vi "ClassifyRX.vi"(8 "error in (no error)":errorcluster, 10 "msg to Log":string, 11 "Log in":refnum<class "Log.lvclass">) -> (0 "error out":errorcluster, 3 "Log out":refnum<class "Log.lvclass">)   [LabVIEW 2018, in "Log.lvclass"]
uses:
  Log.lvclass
  Log.lvclass/Log.ctl
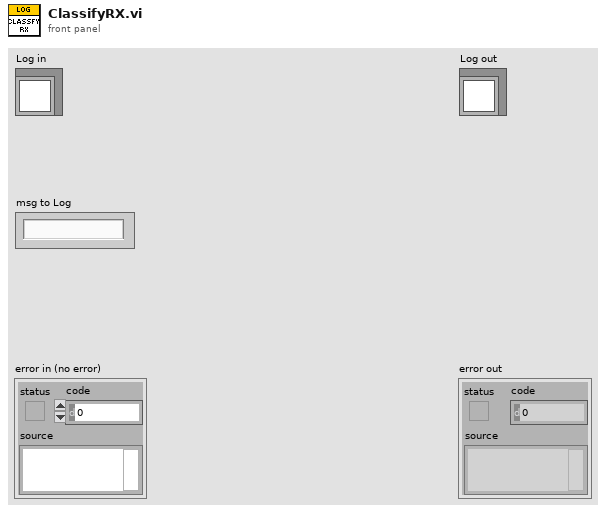
[diagram p1: front panel]
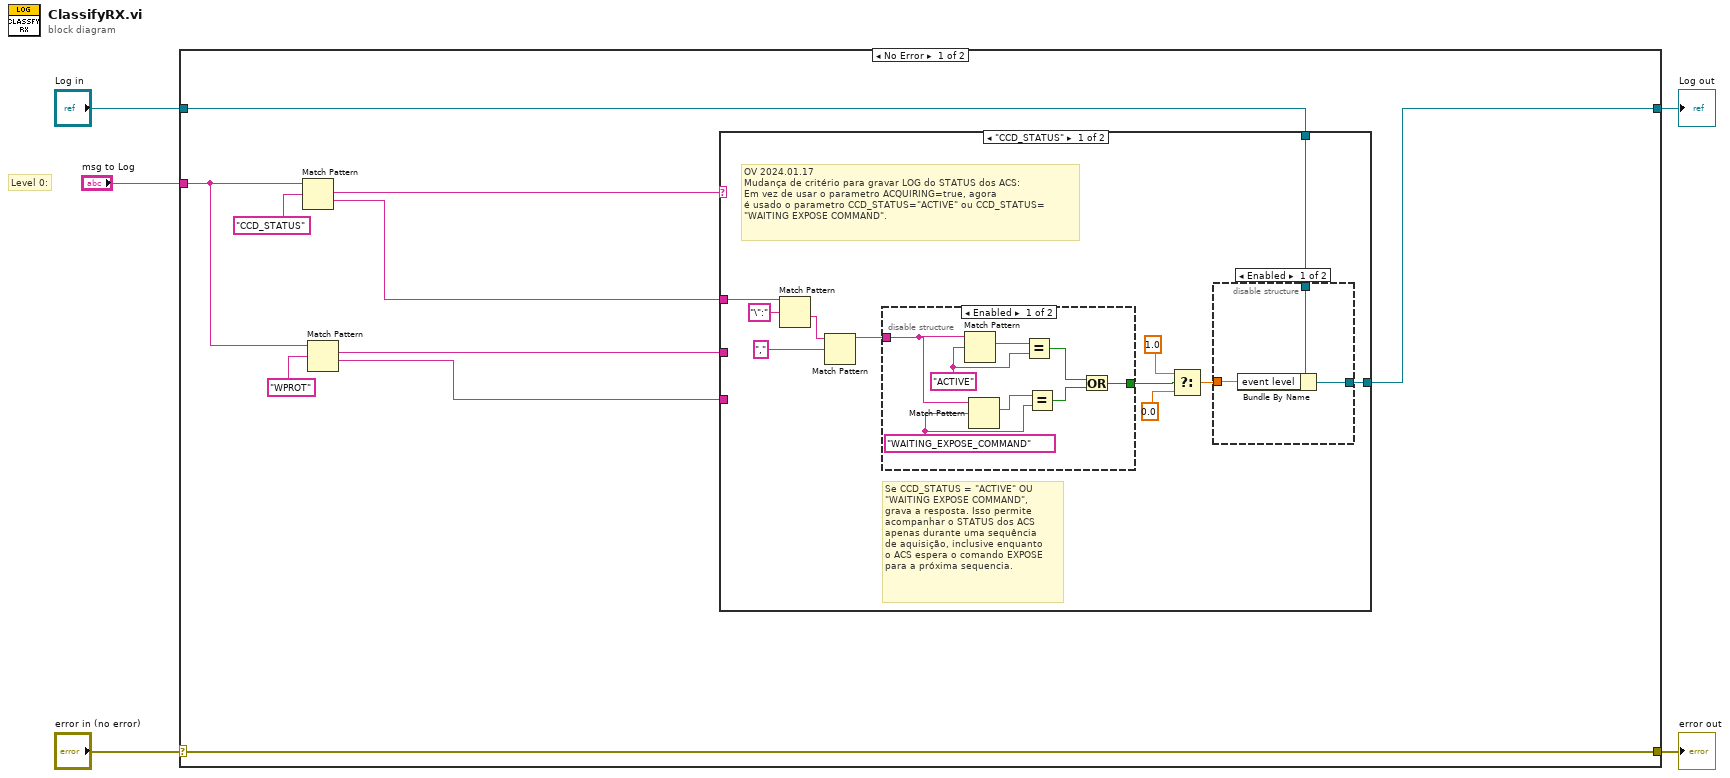
[diagram p0: block diagram]
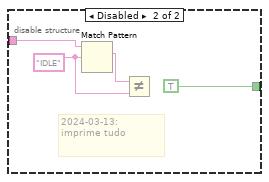
[diagram p2: hidden frame]
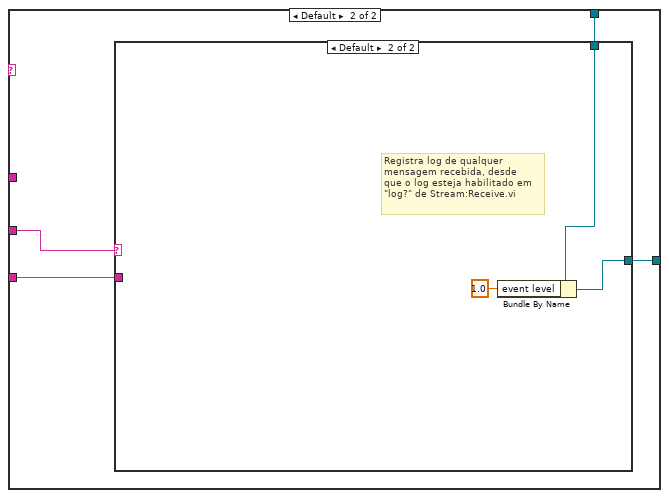
[diagram p4: hidden frame]
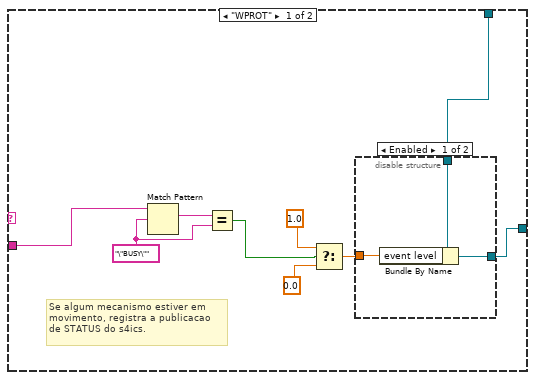
[diagram p5: hidden frame]
diagram:
  # "Level 0:"
  n1 = case shown="No Error" "error in (no error)" {
    selector: "error in (no error)" -> [w15 w64]
    tunnel: [w15 w64] -> w4
    tunnel: [w12 w63] -> w2
    tunnel: "Log in" -> [w13 w63]
    tunnel: "msg to Log" -> [w8 _]
    frame No Error {
      n2 = Match Pattern(string=w8, regular expression="CCD_STATUS") -> (match substring=w11:string, after substring=w10:string)  [unwired: 1 in, 2 out]
      n3 = Match Pattern(string=w8, regular expression="WPROT") -> (match substring=w7:string, after substring=w6:string)  [unwired: 1 in, 2 out]
      n4 = case shown="\"CCD_STATUS\"" w11 {
        tunnel: w13 -> [w26 w46]
        tunnel: [w25 w45] -> w12
        tunnel: w10 -> [w24 _]
        tunnel: w7 -> [_ w44]
        tunnel: w6 -> [_ w43]
        frame "CCD_STATUS" {
          # "OV 2024.01.17\nMudança de critério para gravar LOG do STATUS dos ACS:\nEm vez de usar o parametro ACQUIRING=true, agora\né usado o parametro CCD_STATUS=\"ACTIVE\" ou CCD_STATUS=\n\"WAITING EXPOSE COMMAND\"."
          # "Se CCD_STATUS = \"ACTIVE\" OU \n\"WAITING EXPOSE COMMAND\", \ngrava a resposta. Isso permite \nacompanhar o STATUS dos ACS \napenas durante uma sequência \nde aquisição, inclusive enquanto \no ACS espera o comando EXPOSE\npara a próxima sequencia."
          n5 = Match Pattern(string=w24, regular expression="\":") -> (after substring=w22:string)  [unwired: 1 in, 3 out]
          n6 = Match Pattern(string=w22, regular expression=",") -> (before substring=w18:string)  [unwired: 1 in, 3 out]
          n7 = disable-structure shown="Enabled" {
            disable-tunnel: [w34 TRUE] -> w19
            disable-tunnel: w18 -> [w31 w38]
            frame Enabled {
              w29 = "WAITING_EXPOSE_COMMAND"
              w32 = "ACTIVE"
              n8 = Match Pattern(string=w31, regular expression=w32) -> (match substring=w33:string)  [unwired: 1 in, 3 out]
              n9 = Match Pattern(string=w31, regular expression=w29) -> (match substring=w30:string)  [unwired: 1 in, 3 out]
              n10 = Equal?(x=w33, y=w32) -> (x = y?=w28:bool)
              n11 = Equal?(x=w30, y=w29) -> (x = y?=w27:bool)
              n12 = Or(x=w28, y=w27) -> (x .or. y?=w34:bool)
            }
            frame Disabled {
              w36 = "IDLE"
              # "2024-03-13:\nimprime tudo"
              n13 = Match Pattern(string=w38, regular expression=w36) -> (match substring=w37:string)  [unwired: 1 in, 3 out]
              n14 = Not Equal?(x=w37, y=w36) -> ()  [unwired: 1 out]
            }
          }
          n15 = Select(t=1.0 ("current level"), s=w19, f=0.0) -> (s? t:f=w20:dbl)
          n16 = disable-structure shown="Enabled" {
            disable-tunnel: w26 -> [w41 w42]
            disable-tunnel: [w40 w42] -> w25
            disable-tunnel: w20 -> [w39 _]
            frame Enabled {
              n17 = Bundle By Name(cluster=w41, "event level"=w39) -> (w40:refnum<class "Log.lvclass">)
            }
            frame Disabled {
            }
          }
        }
        frame Default {
          n18 = case shown="Default" w44 {
            tunnel: w46 -> [w49 w62]
            tunnel: [w48 w61] -> w45
            tunnel: w43 -> [w53 _]
            frame "WPROT" {
              w54 = "\"BUSY\""
              # "Se algum mecanismo estiver em\nmovimento, registra a publicacao\nde STATUS do s4ics."
              n19 = Match Pattern(string=w53, regular expression=w54) -> (match substring=w55:string)  [unwired: 1 in, 3 out]
              n20 = Equal?(x=w55, y=w54) -> (x = y?=w47:bool)
              n21 = Select(t=1.0 ("current level"), s=w47, f=0.0) -> (s? t:f=w52:dbl)
              n22 = disable-structure shown="Enabled" {
                disable-tunnel: w49 -> [w58 w59]
                disable-tunnel: [w57 w59] -> w48
                disable-tunnel: w52 -> [w56 _]
                frame Enabled {
                  n23 = Bundle By Name(cluster=w58, "event level"=w56) -> (w57:refnum<class "Log.lvclass">)
                }
                frame Disabled {
                }
              }
            }
            frame Default {
              # "Registra log de qualquer\nmensagem recebida, desde\nque o log esteja habilitado em\n\"log?\" de Stream:Receive.vi"
              n24 = Bundle By Name(cluster=w62, "event level"=1.0) -> (w61:refnum<class "Log.lvclass">)
            }
          }
        }
      }
    }
    frame Error {
    }
  }
  "error out" <- w4
  "Log out" <- w2
